vi "cameraExtTrigger_writeToHardDrive.vi"() -> ()   [LabVIEW 2015]
panel:
  in  "File":path=path "C:/Users/sims01/Desktop/triggering1711/imgStack"
  in  "noFrames":i32=10
  out "Frame Count":i32=1
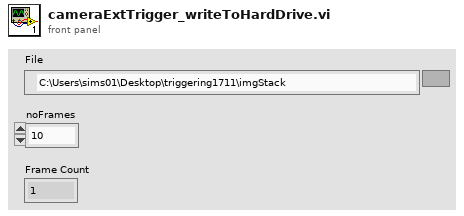
[diagram p1: front panel]
types:
  T1 = cluster{"Mode":u32, "Polarity":u32, "Times":u32, "Delay":dbl}
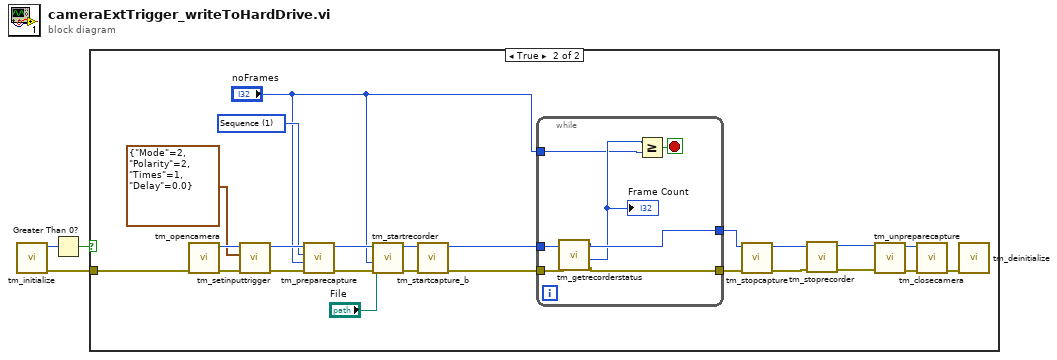
[diagram p0: block diagram]
diagram:
  n1 = call <userlib>:"tm_initialize.vi"() -> ("error out"=w3:errorcluster, "Number Of Cameras"=w1:u32)  [unwired: 8 in, 2 out]
  n2 = Greater Than 0?(x=w1) -> (x > 0?=w2:bool)
  n3 = case shown="True" w2 {
    tunnel: w3 -> [_ w27]
    frame False {
    }
    frame True {
      w23 = 1 items=["Snap", "Sequence"] ("Capture mode")
      n4 = call <userlib>:"tm_opencamera.vi"("error in (no error)"=w27) -> ("error out"=w18:errorcluster, "Handle out"=w26:u32)  [unwired: 8 in, 1 out]
      n5 = call <userlib>:"tm_setinputtrigger.vi"("error in (no error)"=w18, "Parameters"=T1 {"Mode"=2, "Polarity"=2, "Times"=1, "Delay"=0.0}, "Handle in"=w26) -> ("error out"=w17:errorcluster, "Handle out"=w24:u32)  [unwired: 7 in]
      n6 = call <userlib>:"tm_preparecapture.vi"("error in (no error)"=w17, "Frames"="noFrames", "Capture mode"=w23, "Handle in"=w24) -> ("error out"=w12:errorcluster, "Handle out"=w13:u32)  [unwired: 4 in, 2 out]
      n7 = call <userlib>:"tm_startrecorder.vi"("error in (no error)"=w12, "frames"="noFrames", "File"="File", "Handle in"=w13) -> ("error out"=w14:errorcluster, "Handle out"=w15:u32)  [unwired: 6 in]
      n8 = call <userlib>:"tm_startcapture_b.vi"("error in (no error)"=w14, "Handle in"=w15) -> ("error out"=w10:errorcluster, "Handle out"=w11:u32)  [unwired: 8 in]
      n9 = while {
        tunnel: "noFrames" -> [w29]
        tunnel: [w32] -> w20
        tunnel: [w31] -> w16
        tunnel: w11 -> [w34]
        tunnel: w10 -> [w33]
        stop <- w28 stop-if-true
        n10 = call <userlib>:"tm_getrecorderstatus.vi"("error in (no error)"=w33, "Handle"=w34) -> ("error out"=w31:errorcluster, "Count"=w30:i32, "Handle"=w32:u32)  [unwired: 6 in, 1 out]
        "Frame Count" <- w30
        n11 = Greater Or Equal?(x=w30, y=w29) -> (x >= y?=w28:bool)
      }
      n12 = call <userlib>:"tm_stopcapture.vi"("error in (no error)"=w16, "Handle in"=w20) -> ("error out"=w8:errorcluster, "Handle out"=w9:u32)  [unwired: 8 in]
      n13 = call <userlib>:"tm_stoprecorder.vi"("error in (no error)"=w8, "Handle in"=w9) -> ("error out"=w6:errorcluster, "Handle out"=w7:u32)  [unwired: 8 in]
      n14 = call <userlib>:"tm_unpreparecapture.vi"("error in (no error)"=w6, "Handle in"=w7) -> ("error out"=w21:errorcluster, "Handle out"=w19:u32)  [unwired: 8 in]
      n15 = call <userlib>:"tm_closecamera.vi"("error in (no error)"=w21, "Handle in"=w19) -> ("error out"=w22:errorcluster)  [unwired: 9 in]
      n16 = call <userlib>:"tm_deinitialize.vi"("error in (no error)"=w22) -> ()  [unwired: 10 in, 1 out]
    }
  }
